vi "RS232.vi"() -> ()   [LabVIEW 2014]
uses:
  <vilib>/Instr/_visa.llb/VISA Configure Serial Port (Instr).vi
panel:
  out "element":u8
  in  "stop":bool
  in  "VISA resource name":refnum<visa-resource-name>
  in  "write buffer":string
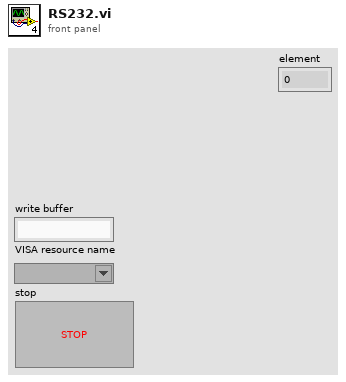
[diagram p1: front panel]
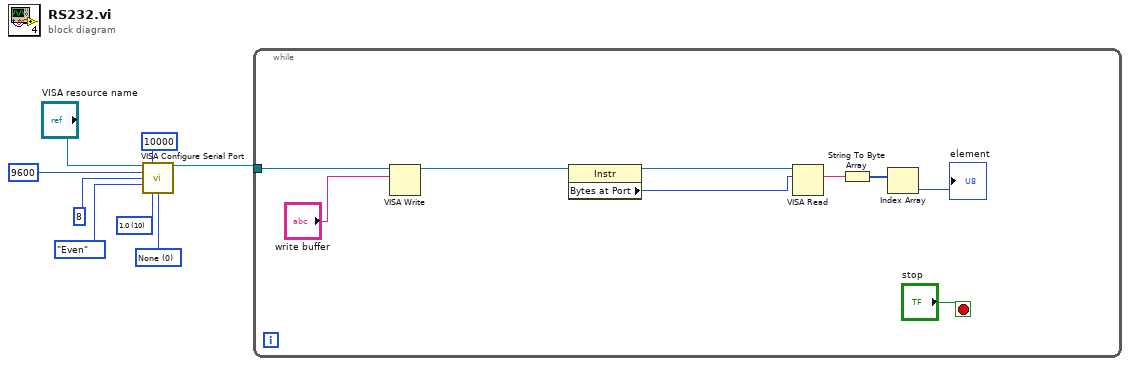
[diagram p0: block diagram]
diagram:
  w1 = u16 0 items=["None", "XON/XOFF", "RTS/CTS", "XON/XOFF & RTS/CTS", "DTR/DSR", "XON/XOFF & DTR/DSR"] ("flow control (0:none)")
  w2 = u16 10 items=["1.0"=10, "1.5"=15, "2.0"=20] ("stop bits (10: 1 bit)")
  n1 = call-poly "VISA Configure Serial Port"("VISA resource name"="VISA resource name", "timeout (10sec)"=u32 10000, "baud rate (9600)"=u32 9600, "data bits (8)"=u16 8, "parity (0:none)"=enum16{"None", "Odd", "Even", "Mark", "Space"}."Even", "stop bits (10: 1 bit)"=w2, "flow control (0:none)"=w1) -> ("VISA resource name out"=w8:refnum<visa-resource-name>)  [unwired: 7 in, 1 out]
  n2 = while {
    tunnel: w8 -> [w13]
    stop <- "stop" stop-if-true
    n3 = VISA Write(VISA resource name=w13, write buffer="write buffer") -> (VISA resource name out=w17:refnum<visa-resource-name>)  [unwired: 1 in, 2 out]
    n4 = property class="Instr"(reference=w17) -> (reference out=w16:refnum<visa-resource-name>, "Bytes at Port"=w15:u32)  [unwired: 1 in, 1 out]
    n5 = VISA Read(VISA resource name=w16, byte count=w15) -> (read buffer=w11:string)  [unwired: 1 in, 3 out]
    n6 = String To Byte Array(string=w11) -> (unsigned byte array=w10:u8[])
    n7 = Index Array(array=w10) -> (element=→"element":u8)  [unwired: 1 in]
  }
